vi "Bomba.vi"() -> ()   [LabVIEW 2020]
uses:
  <vilib>/Instr/_visa.llb/VISA Configure Serial Port (Instr).vi
panel:
  in  "Boolean":bool
  out "concatenated string":string
  out "F-format string":string
  in  "Slide":u8(slide) scale=0.0..255.0
  out "return count":u32
  out "error out":errorcluster
  in  "stop":bool
  in  "VISA resource name":refnum<visa-resource-name>
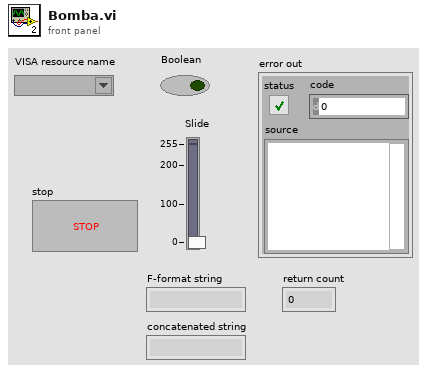
[diagram p1: front panel]
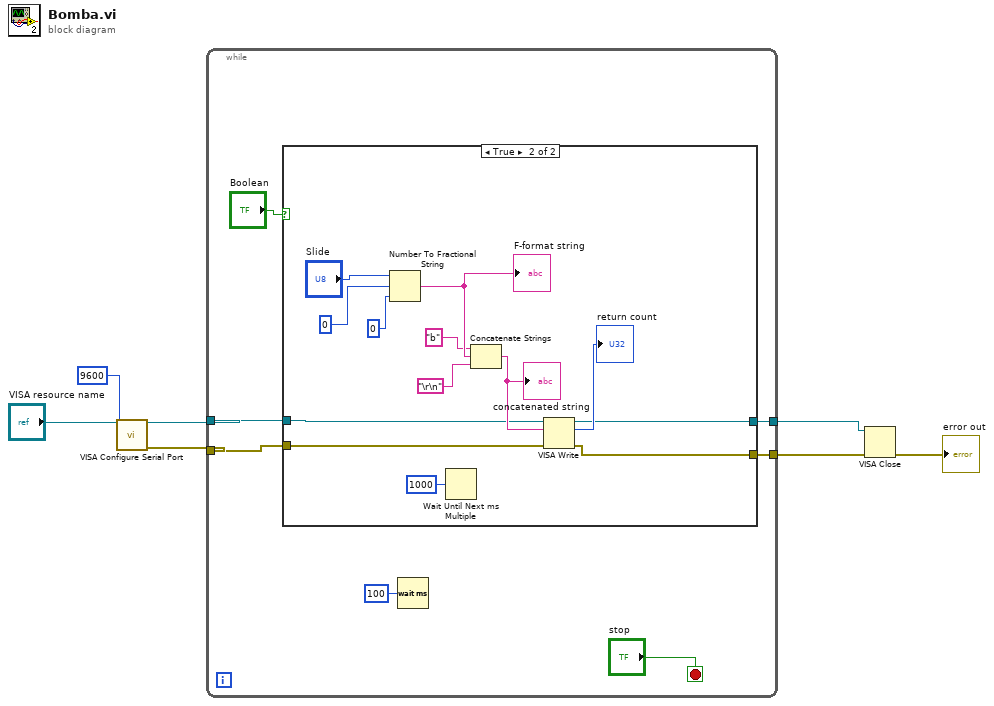
[diagram p0: block diagram]
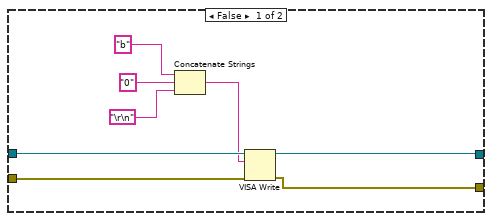
[diagram p2: hidden frame]
diagram:
  n1 = call-poly "VISA Configure Serial Port"("VISA resource name"="VISA resource name", "baud rate (9600)"=u32 9600) -> ("VISA resource name out"=w5:refnum<visa-resource-name>, "error out"=w4:errorcluster)  [unwired: 12 in]
  n2 = while {
    tunnel: w5 -> [w12]
    tunnel: w4 -> [w11]
    tunnel: [w10] -> w2
    tunnel: [w9] -> w1
    stop <- "stop" stop-if-true
    n3 = case shown="True" "Boolean" {
      tunnel: w12 -> [w22 w26]
      tunnel: w11 -> [w21 w27]
      tunnel: [w19 w25] -> w10
      tunnel: [w20 w24] -> w9
      frame False {
        n4 = Concatenate Strings("b" ("string"), "0" ("string"), "\r\n") -> (w16:string)
        n5 = VISA Write(VISA resource name=w22, write buffer=w16, error in (no error)=w21) -> (VISA resource name out=w19:refnum<visa-resource-name>, error out=w20:errorcluster)  [unwired: 1 out]
      }
      frame True {
        n6 = Number To Fractional String(number="Slide", width (-)=i16 0, precision (6)=i16 0) -> (F-format string=w29:string)  [unwired: 1 in]
        "F-format string" <- w29
        n7 = Wait Until Next ms Multiple(millisecond multiple=u32 1000) -> ()  [unwired: 1 out]
        n8 = Concatenate Strings("b" ("string"), w29, "\r\n") -> (w34:string)
        "concatenated string" <- w34
        n9 = VISA Write(VISA resource name=w26, write buffer=w34, error in (no error)=w27) -> (VISA resource name out=w25:refnum<visa-resource-name>, return count=→"return count":u32, error out=w24:errorcluster)
      }
    }
    n10 = Wait (ms)(milliseconds to wait=u32 100) -> ()  [unwired: 1 out]
  }
  n11 = VISA Close(VISA resource name=w2, error in (no error)=w1) -> (error out=→"error out":errorcluster)
